vi "PRL QUEUE Multiple Elements.vi"(8 "error in":errorcluster, 10 "Elements to Add":string[](array[string]), 11 "queue":refnum<queue>) -> (0 "error out":errorcluster, 3 "queue out":refnum<queue>)   [LabVIEW 2013, in "PMU Recorder Light.lvlib"]
uses:
  PMU Recorder Light.lvlib
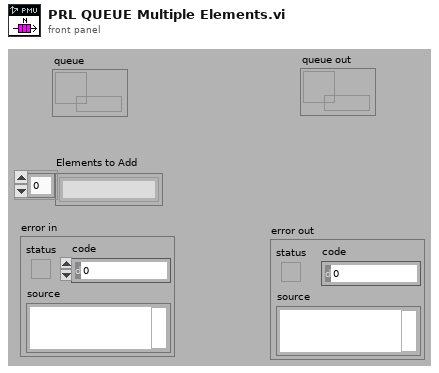
[diagram p1: front panel]
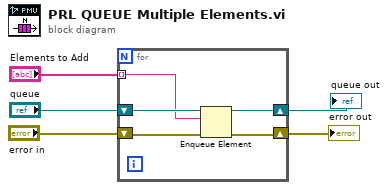
[diagram p0: block diagram]
diagram:
  n1 = for {
    tunnel: "Elements to Add" -> [w9] mode=indexing
    shift-right: [w7] -> w2
    shift-left: "error in" -> [w8]
    shift-right: [w6] -> w1
    shift-left: "queue" -> [w10]
    n2 = Enqueue Element(queue=w10, element=w9, error in (no error)=w8) -> (queue out=w6:refnum<queue>, error out=w7:errorcluster)  [unwired: 2 out]
  }
  "error out" <- w2
  "queue out" <- w1
